vi "Get Config Path.vi"(8 "error in (no error)":errorcluster, 11 "Sys Def Path":path) -> (0 "error out":errorcluster, 3 "Config Path":path)   [LabVIEW 2015]
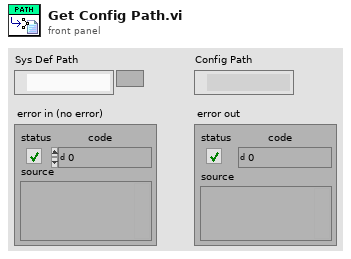
[diagram p1: front panel]
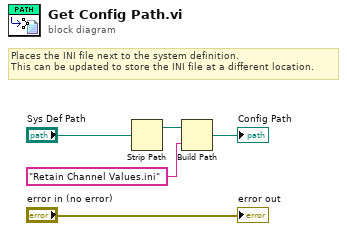
[diagram p0: block diagram]
diagram:
  # "Places the INI file next to the system definition.\nThis can be updated to store the INI file at a different location."
  n1 = Strip Path(path="Sys Def Path") -> (stripped path=w5:path)  [unwired: 1 out]
  n2 = Build Path(base path=w5, name or relative path="Retain Channel Values.ini") -> (appended path=→"Config Path":path)
  "error out" <- "error in (no error)"
